vi "Handle Errors.vi"(8 "error in":errorcluster, 11 "cPAS in":refnum<class "cPAS.lvclass">) -> (0 "error out":errorcluster, 2 "errors":errorcluster[](array[cluster]), 3 "cPAS out":refnum<class "cPAS.lvclass">)   [LabVIEW 2015, in "cPAS.lvclass"]
doc: "Handle errors thrown by the data acquisition system. Most can be thrown out with no deleterious effect on performance - simply report them via whatever means provided by the current instance of the PAS class. If a data acquisition error is thrown however, make sure that the tasks associated with these are restarted to avoid more errors down the line."
uses:
  cPAS.lvclass
  cPAS.lvclass/cPAS.ctl
  Reusable/PAS/Main/PAS.lvclass
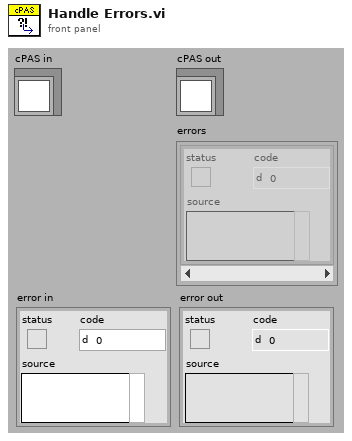
[diagram p1: front panel]
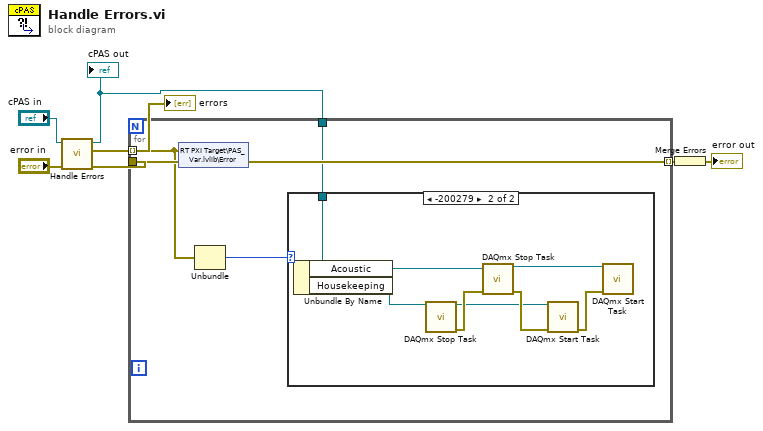
[diagram p0: block diagram]
diagram:
  n1 = call-parent "Handle Errors.vi"("error in"="error in", "Instrument in"="cPAS in") -> ("error out"=w2:errorcluster, "errors"=w3:errorcluster[], "Instrument out"=w1:refnum<class "cPAS.lvclass">)  [unwired: 7 in]
  "cPAS out" <- w1
  "errors" <- w3
  n2 = for {
    tunnel: w3 -> [w10] mode=indexing
    tunnel: w2 -> [w12]
    tunnel: [w11] -> w5 mode=indexing
    tunnel: w1 -> [w8]
    n3 = shared-variable "RT PXI Target\\PAS_Var.lvlib\\Error"(w10, error in=w12) -> (error out=w11:errorcluster)
    n4 = Unbundle(w10) -> ("code"=w9:i32)  [unwired: 2 out]
    n5 = case shown="-200279" w9 {
      tunnel: w8 -> [_ w20]
      frame 0, Default {
      }
      frame -200279 {
        n6 = Unbundle By Name(w20) -> ("Acoustic"=w18:refnum<k21>, "Housekeeping"=w19:refnum<k21>)
        n7 = call <vilib>:"DAQmx Stop Task.vi"("task/channels in"=w19) -> ("task out"=w15:refnum<k21>, "error out"=w17:errorcluster)  [unwired: 13 in]
        n8 = call <vilib>:"DAQmx Stop Task.vi"("task/channels in"=w18, "error in"=w17) -> ("task out"=w14:refnum<k21>, "error out"=w16:errorcluster)  [unwired: 12 in]
        n9 = call <vilib>:"DAQmx Start Task.vi"("task/channels in"=w15, "error in"=w16) -> ("error out"=w13:errorcluster)  [unwired: 12 in, 1 out]
        n10 = call <vilib>:"DAQmx Start Task.vi"("task/channels in"=w14, "error in"=w13) -> ()  [unwired: 12 in, 2 out]
      }
    }
  }
  n11 = Merge Errors(w5) -> (→"error out":errorcluster)
